vi "Modbus Error Checker.vi"(6 "Modbus Configuration":T1, 8 "error in":errorcluster, 11 "Modbus Master in":refnum<class "Modbus Master.lvclass">) -> (0 "error out":errorcluster, 2 "Error Handled":bool, 3 "Modbus Master out":refnum<class "Modbus Master.lvclass">)   [LabVIEW 2018, in "AE75TX Actor.lvlib" / "AE75TX.lvclass"]
uses:
  AE75TX.lvclass
  Controls/Modbus Configuration Cluster.ctl
  <vilib>/ORNL/CSEISMIC DDS/CSEISMIC DDS Base/Data Types/Controls/DeviceID.ctl
  <vilib>/Modbus/master/Modbus Master.lvclass
  <vilib>/Modbus/master/Create Master Instance (TCP).vi
  <vilib>/ORNL/CSEISMIC DDS/CSEISMIC DDS Base/CSEISMIC DDS.lvclass
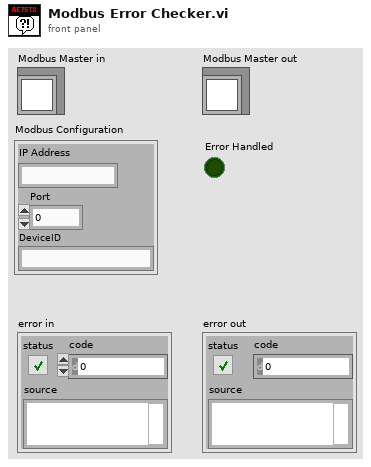
[diagram p1: front panel]
types:
  T1 = typedef "AE75TX Actor.lvlib/AE75TX.lvclass/Modbus Configuration Cluster.ctl" = cluster{"IP Address":string, "Port":u16, "DeviceID":T2}
  T2 = typedef "CSEISMIC DDS.lvlib/CSEISMIC DDS.lvclass/DeviceID.ctl" = string
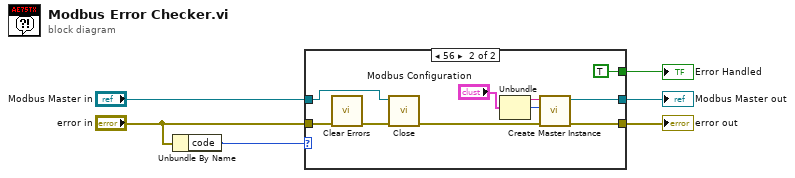
[diagram p0: block diagram]
diagram:
  n1 = Unbundle By Name("error in") -> ("code"=w2:i32)
  n2 = case shown="56" w2 {
    tunnel: "error in" -> [w8 w18]
    tunnel: [w8 w15] -> w4
    tunnel: [w7 w16] -> w5
    tunnel: "Modbus Master in" -> [w7 w17]
    tunnel: [_ TRUE ("Error Handled")] -> w1
    frame 0, Default {
    }
    frame 56 {
      n3 = call <vilib>:"Clear Errors.vi"("error in (no error)"=w18) -> ("error out"=w10:errorcluster)  [unwired: 5 in, 1 out]
      n4 = call-dynamic "Close.vi"("error in (no error)"=w10, "Modbus master in"=w17) -> ("error out"=w14:errorcluster)  [unwired: 9 in]
      n5 = Unbundle("Modbus Configuration") -> ("IP Address"=w12:string, "Port"=w11:u16)  [unwired: 1 out]
      n6 = call-poly <vilib>:"Create Master Instance.vi"("error in (no error)"=w14, "port (502)"=w11, "address"=w12) -> ("error out"=w15:errorcluster, "TCP master instance"=w16:refnum<class "Modbus Master.lvclass">)  [unwired: 7 in]
    }
  }
  "Modbus Master out" <- w5
  "error out" <- w4
  "Error Handled" <- w1
